vi "Test Queues.vi"() -> ()   [LabVIEW 2013]
uses:
  My circular buffer info.ctl
panel:
  in  "command":enum16{"toggle buffers", "data event", "stop"}(ring)
  in  "command 2":enum16{"toggle buffers", "data event", "stop"}(ring)
  out "Command Queue read":string
  in  "stop":bool
  out "read buffer ref queue":refnum<queue>
  out "Event delay queue":refnum<queue>
  out "samples/block/channel 2":i32
  out "number of channels 2":i32
  out "bytes/sample 2":i32
  out "blocks/event":i32
  out "samples/block":i32
  out "num blocks after 2":i32
  out "num blocks  prior 2":i32
  out "xml header":string
  out "archive directory 2":path
  out "buffer2 path 2":path
  out "buffer1 path 2":path
  out "buff ref2":refnum<file>
  out "buff ref1":refnum<file>
  in  "buffer2 path":path
  in  "buffer1 path":path
  in  "archive directory":path
  in  "num blocks  prior":i32
  in  "num blocks after":i32
  in  "bytes/sample":i32
  in  "samples/block/channel":i32
  in  "number of channels":i32
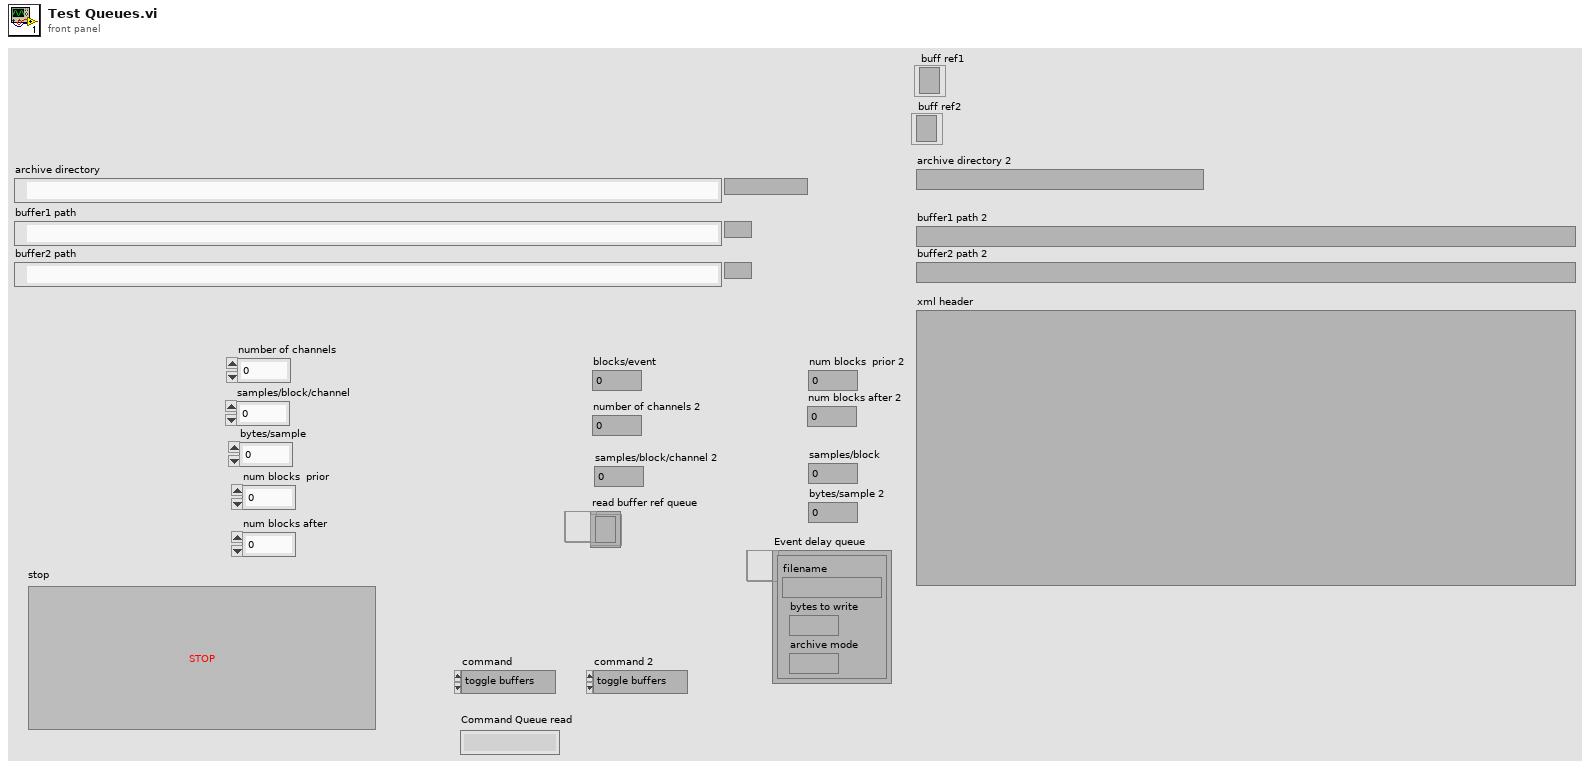
[diagram p1: front panel]
types:
  T1 = typedef "My circular buffer info.ctl" = cluster{"buff ref1":refnum<file>, "buff ref2":refnum<file>, "buffer1 path":path, "buffer2 path":path, "archive directory":path, "xml header":string, "num blocks  prior":i32, "num blocks after":i32, "blocks/event":i32, "samples/block":i32, "bytes/sample":i32, "number of channels":i32, "samples/block/channel":i32, "read buffer ref queue":refnum<queue>, "Event delay queue":refnum<queue>, "command queue":refnum<queue>}
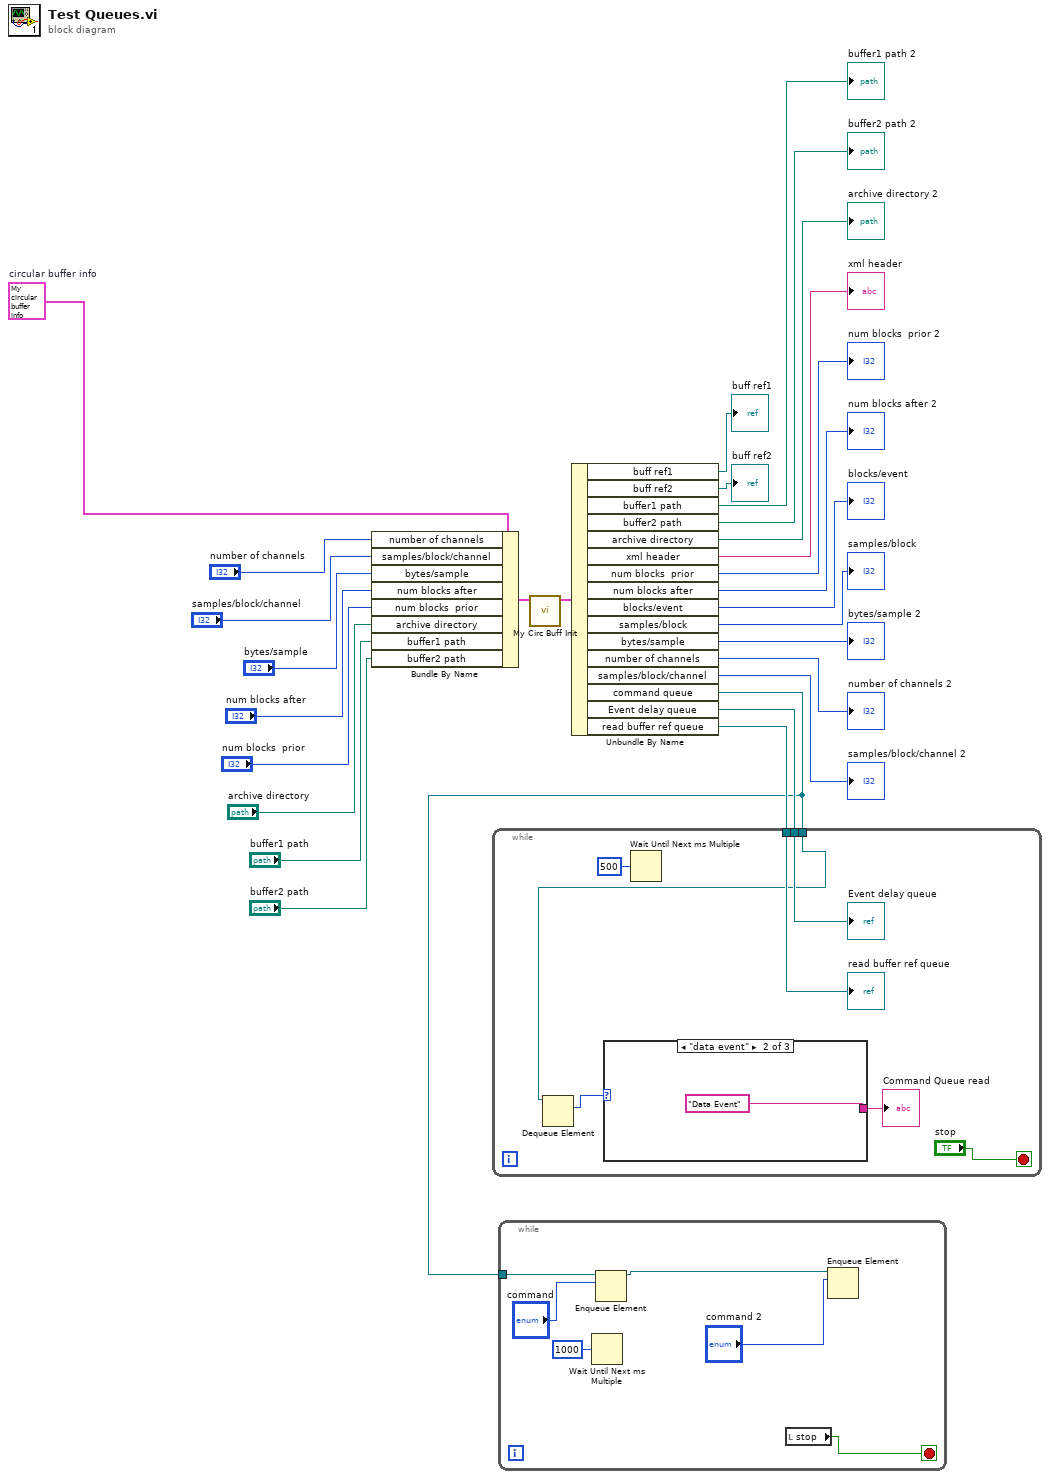
[diagram p0: block diagram]
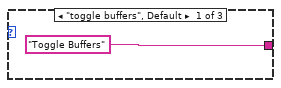
[diagram p2: hidden frame]
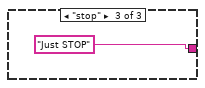
[diagram p3: hidden frame]
diagram:
  w27 = T1 {"buff ref1"=refnum, "buff ref2"=refnum, "buffer1 path"=path "", "buffer2 path"=path "", "archive directory"=path "", "xml header"="", "num blocks  prior"=0, "num blocks after"=0, "blocks/event"=0, "samples/block"=0, "bytes/sample"=0, "number of channels"=0, "samples/block/channel"=0, "read buffer ref queue"=refnum, "Event delay queue"=refnum, "command queue"=refnum}  # circular buffer info
  n1 = Bundle By Name(cluster=w27, "number of channels"="number of channels", "samples/block/channel"="samples/block/channel", "bytes/sample"="bytes/sample", "num blocks after"="num blocks after", "num blocks  prior"="num blocks  prior", "archive directory"="archive directory", "buffer1 path"="buffer1 path", "buffer2 path"="buffer2 path") -> (w18:T1)
  n2 = call "My Circ Buff Init.vi"("circular buffer info"=w18) -> ("circular buffer info out"=w2:T1)  [unwired: 9 in, 1 out]
  n3 = Unbundle By Name(w2) -> ("buff ref1"=→"buff ref1":refnum<file>, "buff ref2"=→"buff ref2":refnum<file>, "buffer1 path"=→"buffer1 path 2":path, "buffer2 path"=→"buffer2 path 2":path, "archive directory"=→"archive directory 2":path, "xml header"=→"xml header":string, "num blocks  prior"=→"num blocks  prior 2":i32, "num blocks after"=→"num blocks after 2":i32, "blocks/event"=→"blocks/event":i32, "samples/block"=→"samples/block":i32, "bytes/sample"=→"bytes/sample 2":i32, "number of channels"=→"number of channels 2":i32, "samples/block/channel"=→"samples/block/channel 2":i32, "command queue"=w1:refnum<queue>, "Event delay queue"=w4:refnum<queue>, "read buffer ref queue"=w3:refnum<queue>)
  n4 = while {
    tunnel: w4 -> [w34]
    tunnel: w3 -> [w33]
    tunnel: w1 -> [w29]
    stop <- "stop" stop-if-true
    n5 = Dequeue Element(queue=w29) -> (element=w31:enum16{"toggle buffers", "data event", "stop"})  [unwired: 2 in, 3 out]
    n6 = case shown="\"data event\"" w31 {
      tunnel: ["Toggle Buffers" ("Command Queue read") "Data Event" ("Command Queue read") "Just STOP" ("Command Queue read")] -> w30
      frame "toggle buffers", Default {
      }
      frame "data event" {
      }
      frame "stop" {
      }
    }
    "Command Queue read" <- w30
    n7 = Wait Until Next ms Multiple(millisecond multiple=u32 500) -> ()  [unwired: 1 out]
    "Event delay queue" <- w34
    "read buffer ref queue" <- w33
  }
  n8 = while {
    tunnel: w1 -> [w41]
    stop <- w42 stop-if-true
    n9 = Wait Until Next ms Multiple(millisecond multiple=u32 1000) -> ()  [unwired: 1 out]
    n10 = Enqueue Element(queue=w41, element="command") -> (queue out=w39:refnum<queue>)  [unwired: 2 in, 2 out]
    n11 = local read "stop"() -> (w42:bool)
    n12 = Enqueue Element(queue=w39, element="command 2") -> ()  [unwired: 2 in, 3 out]
  }
